vi "查询记录.vi"(8 "错误输入":errorcluster, 10 "查询条件":T1, 11 "数据库连接引用 i":T2) -> (0 "error out":errorcluster, 2 "查询结果":string[][](array[string]), 3 "数据库连接引用 o":T2)   [LabVIEW 2017]
uses:
  <vilib>/addons/database/Connection.llb/Conn ObjectReference.ctl
  <vilib>/addons/database/NI_Database_API.lvlib
panel:
  out "字符串数据":string[][](array[string])
  out "sql语句":string
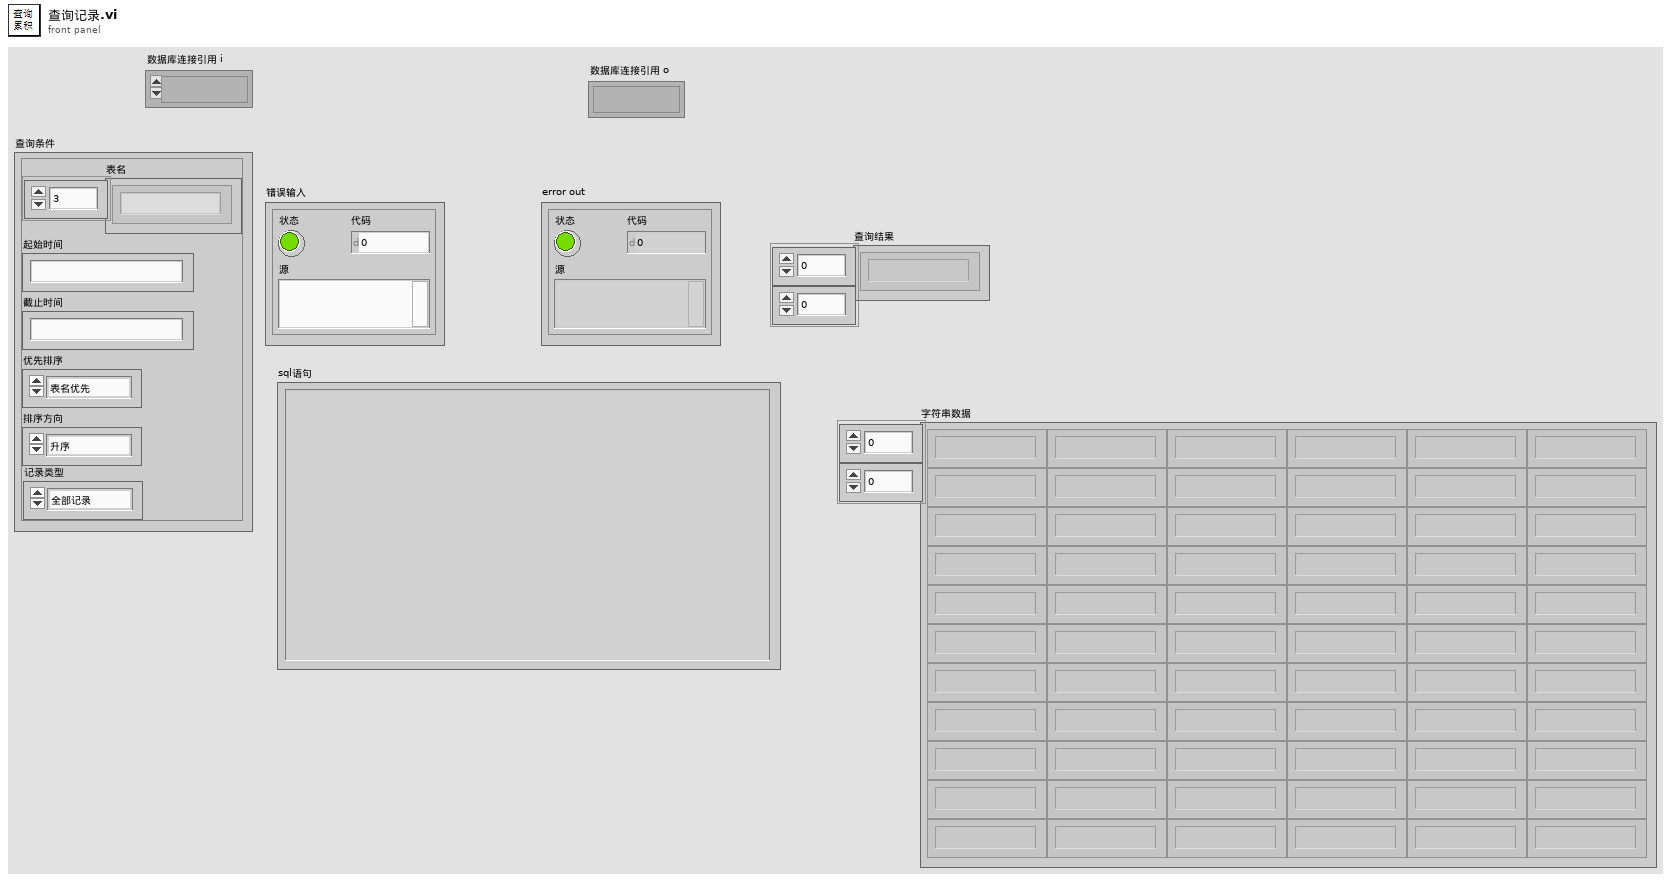
[diagram p1: front panel]
types:
  T1 = cluster{"表名":string[], "起始时间":string, "截止时间":string, "优先排序":enum16{"表名优先", "记录时间优先"}, "排序方向":enum16{"升序", "降序"}, "记录类型":enum16{"全部记录", "报警记录"}}
  T2 = typedef "NI_Database_API.lvlib/Conn ObjectReference.ctl" = refnum<k1>
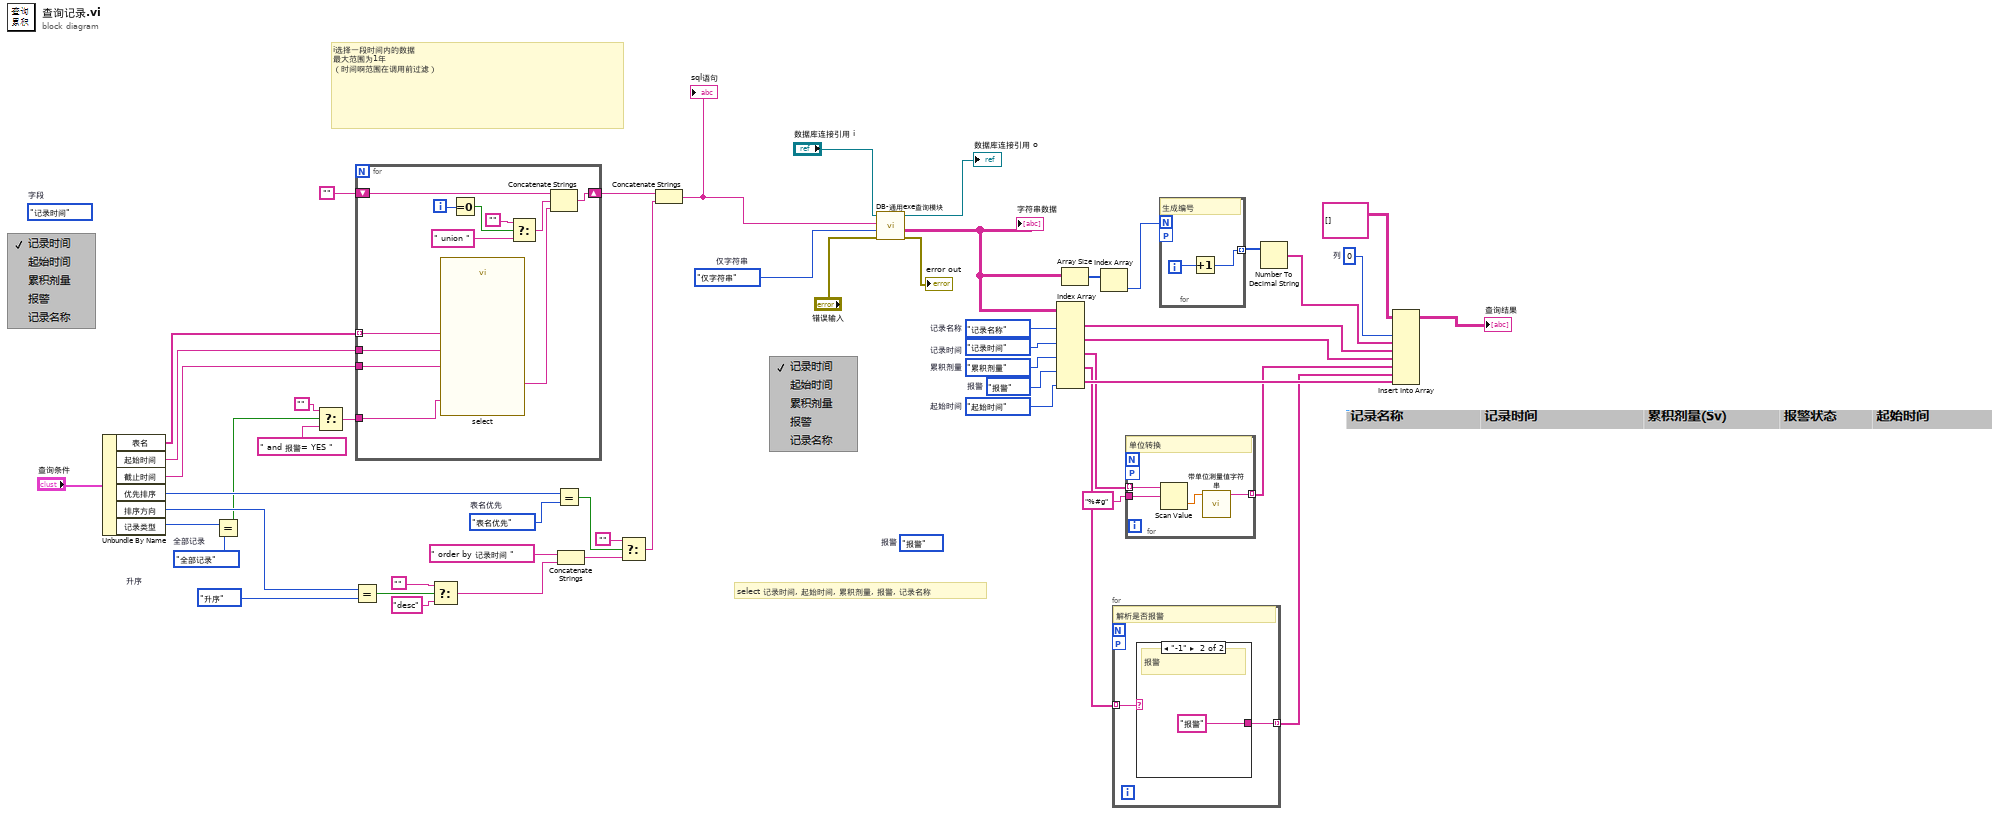
[diagram p0: block diagram]
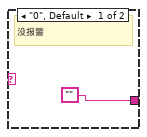
[diagram p2: hidden frame]
diagram:
  w8 = enum16{"全部记录", "报警记录"}."全部记录"  # 全部记录
  w21 = 0  # 列
  (unwired) enum16{"记录时间", "起始时间", "累积剂量", "报警", "记录名称"}."报警"  # 报警
  w27 = enum16{"记录时间", "起始时间", "累积剂量", "报警", "记录名称"}."记录名称"  # 记录名称
  w24 = enum16{"记录时间", "起始时间", "累积剂量", "报警", "记录名称"}."报警"  # 报警
  w25 = enum16{"记录时间", "起始时间", "累积剂量", "报警", "记录名称"}."累积剂量"  # 累积剂量
  w23 = enum16{"记录时间", "起始时间", "累积剂量", "报警", "记录名称"}."起始时间"  # 起始时间
  w26 = enum16{"记录时间", "起始时间", "累积剂量", "报警", "记录名称"}."记录时间"  # 记录时间
  (unwired) enum16{"记录时间", "起始时间", "累积剂量", "报警", "记录名称"}."记录时间"  # 字段
  w31 = enum16{"仅数值", "仅字符串", "数值与字符串"}."仅字符串"  # 仅字符串
  w38 = enum16{"升序", "降序"}."升序"  # 升序
  w46 = enum16{"表名优先", "记录时间优先"}."表名优先"  # 表名优先
  # "select 记录时间, 起始时间, 累积剂量, 报警, 记录名称"
  # "i选择一段时间内的数据\n最大范围为1年\n（时间啊范围在调用前过滤）"
  n1 = Unbundle By Name("查询条件") -> ("表名"=w51:string[], "起始时间"=w50:string, "截止时间"=w49:string, "优先排序"=w47:enum16{"表名优先", "记录时间优先"}, "排序方向"=w39:enum16{"升序", "降序"}, "记录类型"=w9:enum16{"全部记录", "报警记录"})
  n2 = Equal?(x=w9, y=w8) -> (x = y?=w7:bool)
  n3 = Select(t="", s=w7, f=" and 报警= YES ") -> (s? t:f=w4:string)
  n4 = Equal?(x=w39, y=w38) -> (x = y?=w37:bool)
  n5 = for {
    tunnel: w51 -> [w58] mode=indexing
    tunnel: w50 -> [w57]
    tunnel: w49 -> [w56]
    shift-right: [w54] -> w42
    shift-left: "" -> [w55]
    tunnel: w4 -> [w53]
    i -> [w64]
    n6 = call "select"("报警条件"=w53, "表名"=w58, "小时间"=w57, "大时间"=w56) -> ("Result"=w59:string)  [unwired: 10 in, 1 out]
    n7 = Equal To 0?(x=w64) -> (x = 0?=w63:bool)
    n8 = Select(t="", s=w63, f=" union ") -> (s? t:f=w60:string)
    n9 = Concatenate Strings(w55, w60, w59) -> (w54:string)
  }
  n10 = Select(t="", s=w37, f="desc") -> (s? t:f=w34:string)
  n11 = Equal?(x=w47, y=w46) -> (x = y?=w45:bool)
  n12 = Concatenate Strings(" order by 记录时间 ", w34) -> (w40:string)
  n13 = Select(t="", s=w45, f=w40) -> (s? t:f=w41:string)
  n14 = Concatenate Strings(w42, w41) -> (w33:string)
  "sql语句" <- w33
  n15 = call "DB-通用exe查询模块.vi"("error in (no error)"="错误输入", "解析模式"=w31, "SQL query"=w33, "数据库连接引用"="数据库连接引用 i") -> ("error out"=→"error out":errorcluster, "字符串数据"=w14:string[][], "数据库连接引用out"=→"数据库连接引用 o":T2)  [unwired: 3 in, 2 out]
  "字符串数据" <- w14
  n16 = Index Array(array=w14, index (col) #1=w27, index (col) #2=w26, index (col) #3=w25, index (col) #4=w24, index (col) #5=w23) -> (element #1=w20:string[], element #2=w19:string[], element #3=w2:string[], element #4=w16:string[], element #5=w18:string[])  [unwired: 5 in]
  n17 = Array Size(array=w14) -> (size(s)=w13:i32[])
  n18 = Index Array(array=w13) -> (element=w11:i32)  [unwired: 1 in]
  n19 = for {
    tunnel: [w66] -> w15 mode=indexing
    tunnel: w16 -> [w65] mode=indexing
    workers-P: _ -> [_]
    # "解析是否报警"
    n20 = case shown="\"-1\"" w65 {
      tunnel: ["" "报警"] -> w66
      frame "0", Default {
        # "没报警"
      }
      frame "-1" {
        # "报警"
      }
    }
  }
  n21 = for {
    workers-P: _ -> [_]
    tunnel: [w72] -> w3 mode=indexing
    tunnel: w2 -> [w71] mode=indexing
    tunnel: "%#g" ("格式字符串") -> [w69]
    # "单位转换"
    n22 = Scan Value(string=w71, format string=w69) -> (value=w70:dbl)  [unwired: 1 in, 1 out]
    n23 = call "带单位测量值字符串.vi"("测量值"=w70) -> ("结果"=w72:string)  [unwired: 10 in]
  }
  n24 = for {
    N: w11 -> [_]
    tunnel: [w73] -> w12 mode=indexing
    workers-P: _ -> [_]
    i -> [w74]
    # "生成编号"
    n25 = Increment(x=w74) -> (x+1=w73:i32)
  }
  n26 = Number To Decimal String(number=w12) -> (decimal integer string=w10:string[])  [unwired: 1 in]
  n27 = Insert Into Array(array=string[][] [] ("字符串数据"), index (col)=w21, new element #1=w10, new element #2=w20, new element #3=w19, new element #4=w3, new element #5=w15, new element #6=w18) -> (→"查询结果":string[][])  [unwired: 1 in]
